vi "TcpDriver_Init.vi"(11 "response event":T2) -> (2 "Message queue":T1, 3 "TcpDriver out":refnum<class "TcpDriver.lvclass">)   [LabVIEW 2013, in "TcpDriver.lvclass"]
uses:
  TcpDriver.lvclass
  Responder/EventResponder/EventResponder.lvclass
  BaseDriver/BaseDriver.lvclass
  Message/MixerMessage/MixerMessage.lvclass
  driver_status.ctl
  response.ctl
  response_event.ctl
  Message/BaseMessage/BaseMessage.lvclass
  message_queue.ctl
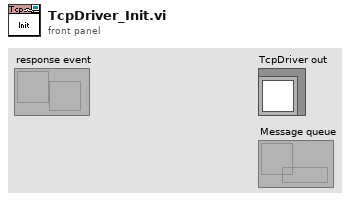
[diagram p1: front panel]
types:
  T1 = typedef "message_queue.ctl" = refnum<queue>
  T2 = typedef "response_event.ctl" = refnum<user-event>
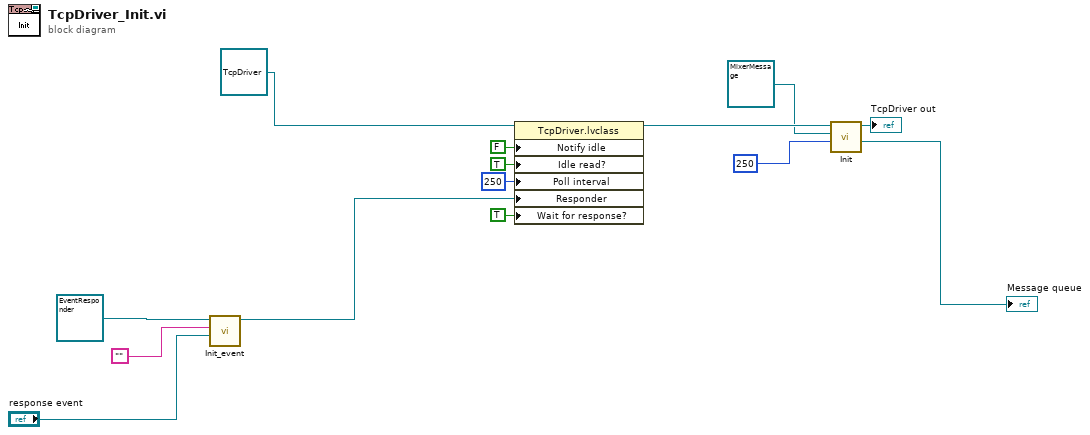
[diagram p0: block diagram]
diagram:
  n1 = call "Init_event.vi"("response event"="response event", "Name"="", "EventResponder in"=refnum<class "EventResponder.lvclass"> refnum) -> ("EventResponder out"=w10:refnum<class "EventResponder.lvclass">)  [unwired: 7 in, 1 out]
  n2 = property class="TcpDriver.lvclass"(reference=refnum<class "TcpDriver.lvclass"> refnum ("TcpDriver.lvclass"), "Notify idle"=FALSE, "Idle read?"=TRUE, "Poll interval"=250, "Responder"=w10, "Wait for response?"=TRUE) -> (reference out=w5:refnum<class "TcpDriver.lvclass">)  [unwired: 1 in, 1 out]
  n3 = call "Init.vi"("Poll interval"=250, "Message type"=refnum<class "MixerMessage.lvclass"> refnum ("MixerMessage.lvclass"), "BaseDriver in"=w5) -> ("Message queue"=→"Message queue":T1, "BaseDriver out"=→"TcpDriver out":refnum<class "TcpDriver.lvclass">)  [unwired: 6 in, 1 out]
